vi "mks670_set_uom.vi"() -> ()   [LabVIEW 2019]
uses:
  ctrl_uom_thcd.ctl
panel:
  in  "uom":T1
  out "Command Read":string
  out "tpg361_visa 3":refnum<visa-resource-name>
  out "err_out 2":errorcluster
  out "Status":bool
  in  "tpg361_b2r":u32
  in  "err_in":errorcluster
  in  "tpg361_delay":u32=500
  in  "tpg361_visa":refnum<visa-resource-name>
  # "VISA"
  # "DELAY"
  # "BYTE AT PORT"
  # "ERROR"
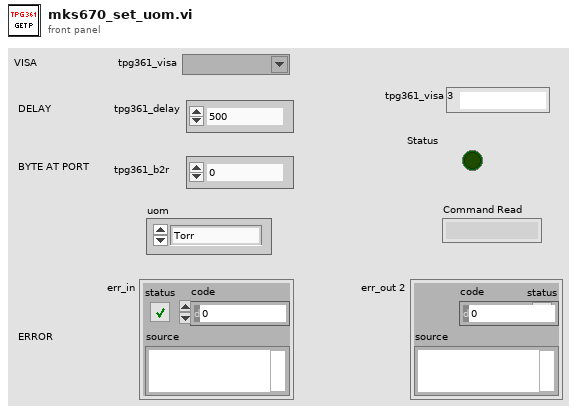
[diagram p1: front panel]
types:
  T1 = typedef "ctrl_uom_thcd.ctl" = enum16{"Torr", "mmHg", "mBar", "pA", "kPA", "psi", "inHG", "in H20", "cm H20", "% fs", "ppm", "mTorr"}
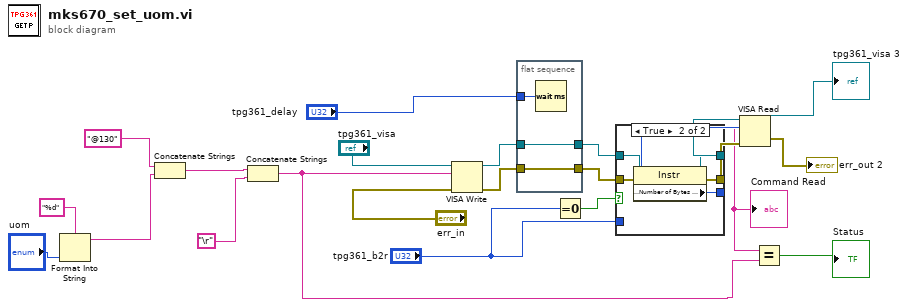
[diagram p0: block diagram]
diagram:
  n1 = Format Into String(format string="%d", "uom") -> (resulting string=w1:string)  [unwired: 2 in, 1 out]
  n2 = Concatenate Strings("@130" ("string"), w1) -> (w2:string)
  n3 = Concatenate Strings(w2, "\r") -> (w5:string)
  n4 = VISA Write(VISA resource name="tpg361_visa", write buffer=w5, error in (no error)="err_in") -> (VISA resource name out=w21:refnum<visa-resource-name>, error out=w23:errorcluster)  [unwired: 1 out]
  n5 = flat-sequence {
    tunnel: w23 -> [w25]
    tunnel: [w25] -> w22
    tunnel: w21 -> [w24]
    tunnel: [w24] -> w20
    tunnel: "tpg361_delay" -> [w26]
    frame #0 {
      n6 = Wait (ms)(milliseconds to wait=w26) -> ()  [unwired: 1 out]
    }
  }
  n7 = Equal To 0?(x="tpg361_b2r") -> (x = 0?=w16:bool)
  n8 = case shown="True" w16 {
    tunnel: w22 -> [w28 w34]
    tunnel: w20 -> [w29 w33]
    tunnel: [w29 w32] -> w14
    tunnel: [w28 w31] -> w13
    tunnel: [w27 w30] -> w12
    tunnel: "tpg361_b2r" -> [w27 _]
    frame False {
    }
    frame True {
      n9 = property class="Instr"(reference=w33, error in=w34) -> (reference out=w32:refnum<visa-resource-name>, error out=w31:errorcluster, "Serial Settings:Number of Bytes at Serial Port"=w30:u32)
    }
  }
  n10 = VISA Read(VISA resource name=w14, byte count=w12, error in (no error)=w13) -> (VISA resource name out=→"tpg361_visa 3":refnum<visa-resource-name>, read buffer=w10:string, error out=→"err_out 2":errorcluster)  [unwired: 1 out]
  "Command Read" <- w10
  n11 = Equal?(x=w10, y=w5) -> (x = y?=→"Status":bool)
